vi "NMRvmefull4.vi"() -> ()   [LabVIEW 2013]
uses:
  <vilib>/Utility/file.llb/Read From Spreadsheet File (DBL).vi
  <vilib>/Analysis/NI_AALBase.lvlib
panel:
  in  "Real/quad Q curve":bool=TRUE
  out "Temperature":dbl(graph)=24.5
  out "+3V supply":dbl=3.026 format="%_4g"
  out "Temp (C)":dbl=24.5 format="%_4g"
  in  "RemovePed":bool=TRUE
  in  "IF / LOG Det":bool
  in  "Q curve file":string="realback213.txt"
  out "File name 2":string="C:\\users\\plm\\Desktop\\rssmt\\realback213.txt"
  in  "AutoBaseline":bool=TRUE
  out "RF OK":bool=TRUE
  out "Peak area (V-MHz)":sgl=0.047207057 format="%.5f"
  in  "Gauss Fit":bool=TRUE
  out "NMR Graph + Fit":cluster{cluster{dbl, "Numeric":dbl}[]}[](graph)=[{[{212.6, "Numeric"=-0.00214345238095235}, {212.60999999999999, "Numeric"=0.006892113095217631}, {212.62, "Numeric"=0.0019276785714510206}, {212.63, "Numeric"=0.006363244047621508}, {212.64, "Numeric"=0.006298809523793053}, {212.65, "Numeric"=-0.00026562499997699607}, {212.66, "Numeric"=0.006969940476195022}, {212.67, "Numeric"=0.010905505952368177}, {212.68, "Numeric"=0.009641071428594498}, {212.69, "Numeric"=0.004676636904768078}, {212.7, "Numeric"=0.0005122023809427875}, {212.71, "Numeric"=-0.00015223214283439923}, {212.72, "Numeric"=-0.008416666666659266}, {212.73, "Numeric"=-0.007381101190482957}, {212.74, "Numeric"=-0.0061455357143089286}, {212.75, "Numeric"=0.0058900297619129925}, {212.76, "Numeric"=0.004725595238090845}, {212.77, "Numeric"=0.003161160714266458}, {212.78, "Numeric"=0.0016967261904848666}, {212.79, "Numeric"=0.0038322916666642705}, {212.8, "Numeric"=-0.0059321428571585295}, {212.81, "Numeric"=-0.008196577380943697}, {212.82, "Numeric"=-0.014061011904762707}, {212.82999999999998, "Numeric"=-0.006825446428580642}, {212.84, "Numeric"=-0.0025898809523726522}, {212.85, "Numeric"=-0.002154315476190119}, {212.85999999999999, "Numeric"=0.0002812499999935124}, {212.87, "Numeric"=-0.00438318452380204}, {212.88, "Numeric"=-0.0012476190476179306}, {212.89, "Numeric"=-0.00021205357143272256}, {212.9, "Numeric"=0.009923511904768166}, {212.91, "Numeric"=0.014159077380953854}, {212.92, "Numeric"=0.02259464285714062}, {212.93, "Numeric"=0.036430208333337974}, {212.94, "Numeric"=0.054065773809525215}, {212.95, "Numeric"=0.10650133928571356}, {212.96, "Numeric"=0.20393690476190737}, {212.97, "Numeric"=0.4019724702380962}, {212.98, "Numeric"=0.5035080357142862}, {212.99, "Numeric"=0.42304360119047385}, {213.0, "Numeric"=0.3538791666666667}, {213.01, "Numeric"=0.33051473214285815}, {213.02, "Numeric"=0.2765502976190475}, {213.03, "Numeric"=0.24828586309523684}, {213.04, "Numeric"=0.25662142857142994}, {213.05, "Numeric"=0.24615699404762076}, {213.06, "Numeric"=0.2482925595238066}, {213.07, "Numeric"=0.23562812500000124}, {213.08, "Numeric"=0.19236369047619362}, {213.09, "Numeric"=0.13109925595237593}, {213.1, "Numeric"=0.09613482142857213}, {213.11, "Numeric"=0.07377038690476609}, {213.12, "Numeric"=0.07290595238094486}, {213.13, "Numeric"=0.05124151785714261}, {213.14000000000001, "Numeric"=0.04147708333333814}, {213.15, "Numeric"=0.031812648809513344}, {213.16, "Numeric"=0.03974821428571268}, {213.17000000000002, "Numeric"=0.0409837797619098}, {213.18, "Numeric"=0.030919345238081458}, {213.19, "Numeric"=0.025954910714282364}, {213.2, "Numeric"=0.01839047619048432}, {213.21, "Numeric"=0.01152604166664914}, {213.22, "Numeric"=0.0018616071428516068}, {213.23, "Numeric"=-0.003102827380944837}, {213.24, "Numeric"=-0.003267261904743482}, {213.25, "Numeric"=-0.009831696428579579}, {213.26, "Numeric"=-0.02009613095237444}, {213.27, "Numeric"=-0.017960565476171506}, {213.28, "Numeric"=-0.013825000000011082}, {213.29, "Numeric"=-0.009389434523804457}, {213.3, "Numeric"=-0.005953869047599914}, {213.31, "Numeric"=-0.001018303571443141}, {213.32, "Numeric"=0.0019172619047652106}, {213.33, "Numeric"=-0.018047172619028776}, {213.34, "Numeric"=-0.013611607142875442}, {213.35, "Numeric"=-0.011976041666665615}, {213.36, "Numeric"=-0.012140476190458018}, {213.37, "Numeric"=-0.005904910714308265}, {213.38, "Numeric"=0.0001306547619031248}, {213.39000000000001, "Numeric"=-0.0015337797618877186}, {213.4, "Numeric"=0.002001785714258554}]}, {[{212.6, "Numeric"=4.776893558475571e-16}, {212.60999999999999, "Numeric"=2.4998938518052677e-15}, {212.62, "Numeric"=1.255832331532795e-14}, {212.63, "Numeric"=6.055860163946861e-14}, {212.64, "Numeric"=2.8032001252118955e-13}, {212.65, "Numeric"=1.245565173214598e-12}, {212.66, "Numeric"=5.31267068658366e-12}, {212.67, "Numeric"=2.1751710942402627e-11}, {212.68, "Numeric"=8.548856700490645e-11}, {212.69, "Numeric"=3.225200648435985e-10}, {212.7, "Numeric"=1.1679910816561408e-09}, {212.71, "Numeric"=4.0602839092061546e-09}, {212.72, "Numeric"=1.3549003796765097e-08}, {212.73, "Numeric"=4.3400268270931275e-08}, {212.74, "Numeric"=1.3344784063174184e-07}, {212.75, "Numeric"=3.938807665763447e-07}, {212.76, "Numeric"=1.1159688835032996e-06}, {212.77, "Numeric"=3.0351033450249673e-06}, {212.78, "Numeric"=7.923717225927055e-06}, {212.79, "Numeric"=1.9857224263191096e-05}, {212.8, "Numeric"=4.77685655501104e-05}, {212.81, "Numeric"=0.00011030620579413602}, {212.82, "Numeric"=0.00024450727185348263}, {212.82999999999998, "Numeric"=0.0005202567224041215}, {212.84, "Numeric"=0.001062619321376955}, {212.85, "Numeric"=0.00208339589052297}, {212.85999999999999, "Numeric"=0.003921028375121005}, {212.87, "Numeric"=0.00708373415515426}, {212.88, "Numeric"=0.012284531843177892}, {212.89, "Numeric"=0.020449799470303114}, {212.9, "Numeric"=0.03267785821490993}, {212.91, "Numeric"=0.05012474792628662}, {212.92, "Numeric"=0.07380485072971074}, {212.93, "Numeric"=0.10431618549469776}, {212.94, "Numeric"=0.141531326388596}, {212.95, "Numeric"=0.1843264006586668}, {212.96, "Numeric"=0.23043932570196038}, {212.97, "Numeric"=0.27654113177117073}, {212.98, "Numeric"=0.318564196067707}, {212.99, "Numeric"=0.35226401239535293}, {213.0, "Numeric"=0.37391568130834746}, {213.01, "Numeric"=0.3809896410966228}, {213.02, "Numeric"=0.37263765937905063}, {213.03, "Numeric"=0.3498600920751344}, {213.04, "Numeric"=0.3153088466879908}, {213.05, "Numeric"=0.2727796658425095}, {213.06, "Numeric"=0.22652801382782384}, {213.07, "Numeric"=0.18057845310601628}, {213.08, "Numeric"=0.13817963040978265}, {213.09, "Numeric"=0.10149770261945476}, {213.1, "Numeric"=0.07156529811815136}, {213.11, "Numeric"=0.048437625424841466}, {213.12, "Numeric"=0.031470039729766065}, {213.13, "Numeric"=0.019626634059215383}, {213.14000000000001, "Numeric"=0.011749745126604191}, {213.15, "Numeric"=0.006752197770040614}, {213.16, "Numeric"=0.003724739884438077}, {213.17000000000002, "Numeric"=0.001972335681903894}, {213.18, "Numeric"=0.0010025355948645779}, {213.19, "Numeric"=0.0004891621640607406}, {213.2, "Numeric"=0.00022910786660302744}, {213.21, "Numeric"=0.00010300569388837138}, {213.22, "Numeric"=4.445458393558479e-05}, {213.23, "Numeric"=1.8416451552346927e-05}, {213.24, "Numeric"=7.3236814655574865e-06}, {213.25, "Numeric"=2.795677209790716e-06}, {213.26, "Numeric"=1.0244215183627779e-06}, {213.27, "Numeric"=3.6033333878935025e-07}, {213.28, "Numeric"=1.2166461504331838e-07}, {213.29, "Numeric"=3.9432854284808336e-08}, {213.3, "Numeric"=1.2268352014433039e-08}, {213.31, "Numeric"=3.663939808945258e-09}, {213.32, "Numeric"=1.0503753455418787e-09}, {213.33, "Numeric"=2.8905121249409887e-10}, {213.34, "Numeric"=7.635529486391247e-11}, {213.35, "Numeric"=1.93614379589947e-11}, {213.36, "Numeric"=4.712703817908686e-12}, {213.37, "Numeric"=1.1011253745842512e-12}, {213.38, "Numeric"=2.469661789025322e-13}, {213.39000000000001, "Numeric"=5.3170688138188436e-14}, {213.4, "Numeric"=1.0988569689482739e-14}]}]
  in  "Amp of Q curve":dbl=3.0 min=0.0 max=7.0 step=0.01 format="%_3f"
  in  "Subtract Q curve":bool=TRUE
  in  "Adjust Tune":bool
  out "Ped Offset":dbl(graph)=0.005645833333333402
  out "Pedestal Difference":dbl(graph)=0.06520833333333734
  out "# Good Spectra":i32=977
  in  "Quality cuts":bool=TRUE
  out "Pedestal OK":bool=TRUE
  out "Sweep #":i32=3604
  out "1st Sweep":bool
  out "ADC volts OK":bool=TRUE
  out "Peak Height Distribution":cluster{"Y":dbl[], "Y":dbl[]}[](graph)=[{"Y"=[0.36242839752414713, 0.3626627543764223, 0.36289711122869756, 0.3631314680809728, 0.363365824933248, 0.3636001817855232, 0.36383453863779847, 0.36406889549007365, 0.3643032523423489, 0.3645376091946241, 0.3647719660468993, 0.36500632289917456, 0.36524067975144975, 0.365475036603725, 0.3657093934560002, 0.3659437503082754, 0.36617810716055066, 0.36641246401282584, 0.3666468208651011, 0.36688117771737633, 0.3671155345696515, 0.36734989142192676, 0.36758424827420194, 0.3678186051264772, 0.3680529619787524, 0.3682873188310276, 0.36852167568330285, 0.3687560325355781, 0.3689903893878533, 0.3692247462401285, 0.3694591030924037, 0.36969345994467895, 0.3699278167969542, 0.3701621736492294, 0.3703965305015046, 0.37063088735377986, 0.37086524420605504, 0.3710996010583303, 0.37133395791060547, 0.3715683147628807, 0.37180267161515596, 0.37203702846743114, 0.3722713853197064, 0.37250574217198157, 0.3727400990242568, 0.37297445587653205, 0.37320881272880724, 0.3734431695810825, 0.3736775264333577, 0.3739118832856329, 0.37414624013790815, 0.37438059699018333, 0.3746149538424586, 0.3748493106947338, 0.375083667547009, 0.37531802439928424, 0.3755523812515595, 0.37578673810383467, 0.3760210949561099, 0.3762554518083851, 0.37648980866066034, 0.3767241655129356, 0.37695852236521077, 0.377192879217486, 0.3774272360697612, 0.37766159292203644, 0.3778959497743117, 0.37813030662658687, 0.3783646634788621, 0.37859902033113735, 0.37883337718341253, 0.3790677340356878, 0.37930209088796296, 0.3795364477402382, 0.37977080459251344, 0.38000516144478863, 0.38023951829706387, 0.3804738751493391, 0.3807082320016143, 0.38094258885388954, 0.3811769457061647, 0.38141130255843997, 0.3816456594107152, 0.3818800162629904, 0.38211437311526564, 0.3823487299675409, 0.38258308681981607, 0.3828174436720913, 0.3830518005243665, 0.38328615737664173, 0.383520514228917, 0.38375487108119216, 0.3839892279334674, 0.3842235847857426, 0.38445794163801783, 0.38469229849029307, 0.38492665534256826, 0.3851610121948435, 0.38539536904711874, 0.3856297258993939], "Y"=[1.0, 0.0, 2.0, 1.0, 3.0, 3.0, 2.0, 1.0, 2.0, 4.0, 0.0, 3.0, 4.0, 3.0, 4.0, 2.0, 3.0, 6.0, 4.0, 4.0, 4.0, 6.0, 11.0, 6.0, 7.0, 6.0, 8.0, 8.0, 6.0, 13.0, 10.0, 12.0, 14.0, 27.0, 14.0, 15.0, 23.0, 16.0, 16.0, 12.0, 13.0, 24.0, 23.0, 17.0, 28.0, 22.0, 18.0, 20.0, 25.0, 21.0, 25.0, 21.0, 24.0, 16.0, 27.0, 16.0, 18.0, 13.0, 18.0, 23.0, 20.0, 19.0, 7.0, 13.0, 16.0, 12.0, 20.0, 15.0, 13.0, 13.0, 9.0, 13.0, 11.0, 10.0, 6.0, 4.0, 10.0, 5.0, 9.0, 6.0, 3.0, 5.0, 5.0, 3.0, 4.0, 3.0, 3.0, 3.0, 3.0, 1.0, 4.0, 2.0, 3.0, 1.0, 1.0, 1.0, 1.0, 1.0, 0.0, 1.0]}]
  in  "# of Sweeps":i32=10000
  out "Std Dev (V)":dbl=0.004257288736008398 format="%_2g"
  out "Peak mean (V)":dbl=0.37397306272927033 format="%_4g"
  out "Peak Height":dbl(graph)=0.38100328829507124
  in  "Raw Data":bool=TRUE
  in  "Tank RF":bool=TRUE
  in  "IF Atten (dB)":i8 min=0 max=31 step=1
  in  "IFoffset (V)":dbl=-2.0905283999999975 min=-4.0 max=4.0 step=0.001 format="%.4f"
  in  "Tune  (V)":dbl=0.6128999999999999 min=0.0 max=5.0 step=0.001 format="%.4f"
  in  "Hi / Lo IF Gain":bool
  out "Voltage Array":sgl[](array[numeric])=[0.449, 0.4352, 0.408, 0.3908, 0.3697, 0.3427, 0.3301, 0.3148, 0.2949, 0.2719, 0.2503, 0.2328, 0.2083, 0.1937, 0.1799, 0.1775, 0.1625, 0.1477, 0.1336, 0.1237, 0.1025, 0.0894, 0.0733, 0.0709, 0.0661, 0.0581, 0.0527, 0.0408, 0.0373, 0.0323, 0.037, 0.0364, 0.0406, 0.0508, 0.0654, 0.1154, 0.211, 0.4078, 0.5087, 0.4282, 0.3596, 0.3374, 0.2852, 0.2593, 0.2706, 0.2637, 0.27, 0.2621, 0.2242, 0.1689, 0.1405, 0.1253, 0.1322, 0.1189, 0.1181, 0.118, 0.1361, 0.1481, 0.1494, 0.1564, 0.1614, 0.1677, 0.1718, 0.1812, 0.196, 0.205, 0.2109, 0.2298, 0.2513, 0.2737, 0.2957, 0.3198, 0.3425, 0.3429, 0.3683, 0.3915, 0.4135, 0.4425, 0.4719, 0.4942, 0.5223] format="%.4f"
  in  "Invert Polarity":bool
  out "Pedestal Diff (V)":sgl=0.06520833 format="%.3f"
  out "Peak amp (V)":sgl=0.3810033 format="%.3f"
  in  "Save Data to File":bool
  in  "RF Level (dBm)":dbl=-1.0 min=-10.0 max=1.0 step=0.1 format="%.2f"
  out "SMT error out":errorcluster
  out "Sample RMS (V)":dbl=0.016388888888888887 format="%.4f"
  in  "# Sample/step":i32=200 min=1 max=1000 step=100
  in  "Step Width (MHz)":dbl=0.01 min=0.0 max=1000.0 step=0.0005 format="%.4f"
  in  "Freq Span (MHz)":dbl=0.8 min=0.0 max=3000.0 step=0.1 format="%.3f"
  in  "Center Freq (MHz)":dbl=213.0 min=0.005 max=6000.0 step=0.1 format="%.3f"
  in  "Sweep Mode":u16(ring)=3 items=["Off", "Single", "Auto", "Step"]
  in  "GPIB Addr (28)":refnum<visa-resource-name>="GPIB0::28::INSTR"
  # "E1039 Prototype NMR Control Panel"
  # "Settings"
  # "D\nA\nC"
  # "R\nF\n\nG\nE\nN \n\n+\n\nI\nF"
  # "A\nD\nC"
  # "D\nA\nT\nA\n\n+\n\nA \nN\nA\nL\nY\nS\nI\nS"
  # "I\n/\nO"
  # "Results"
  # "A\nv\ne\nr\na\ng\ne"
  # "S\nw\ne\ne\np"
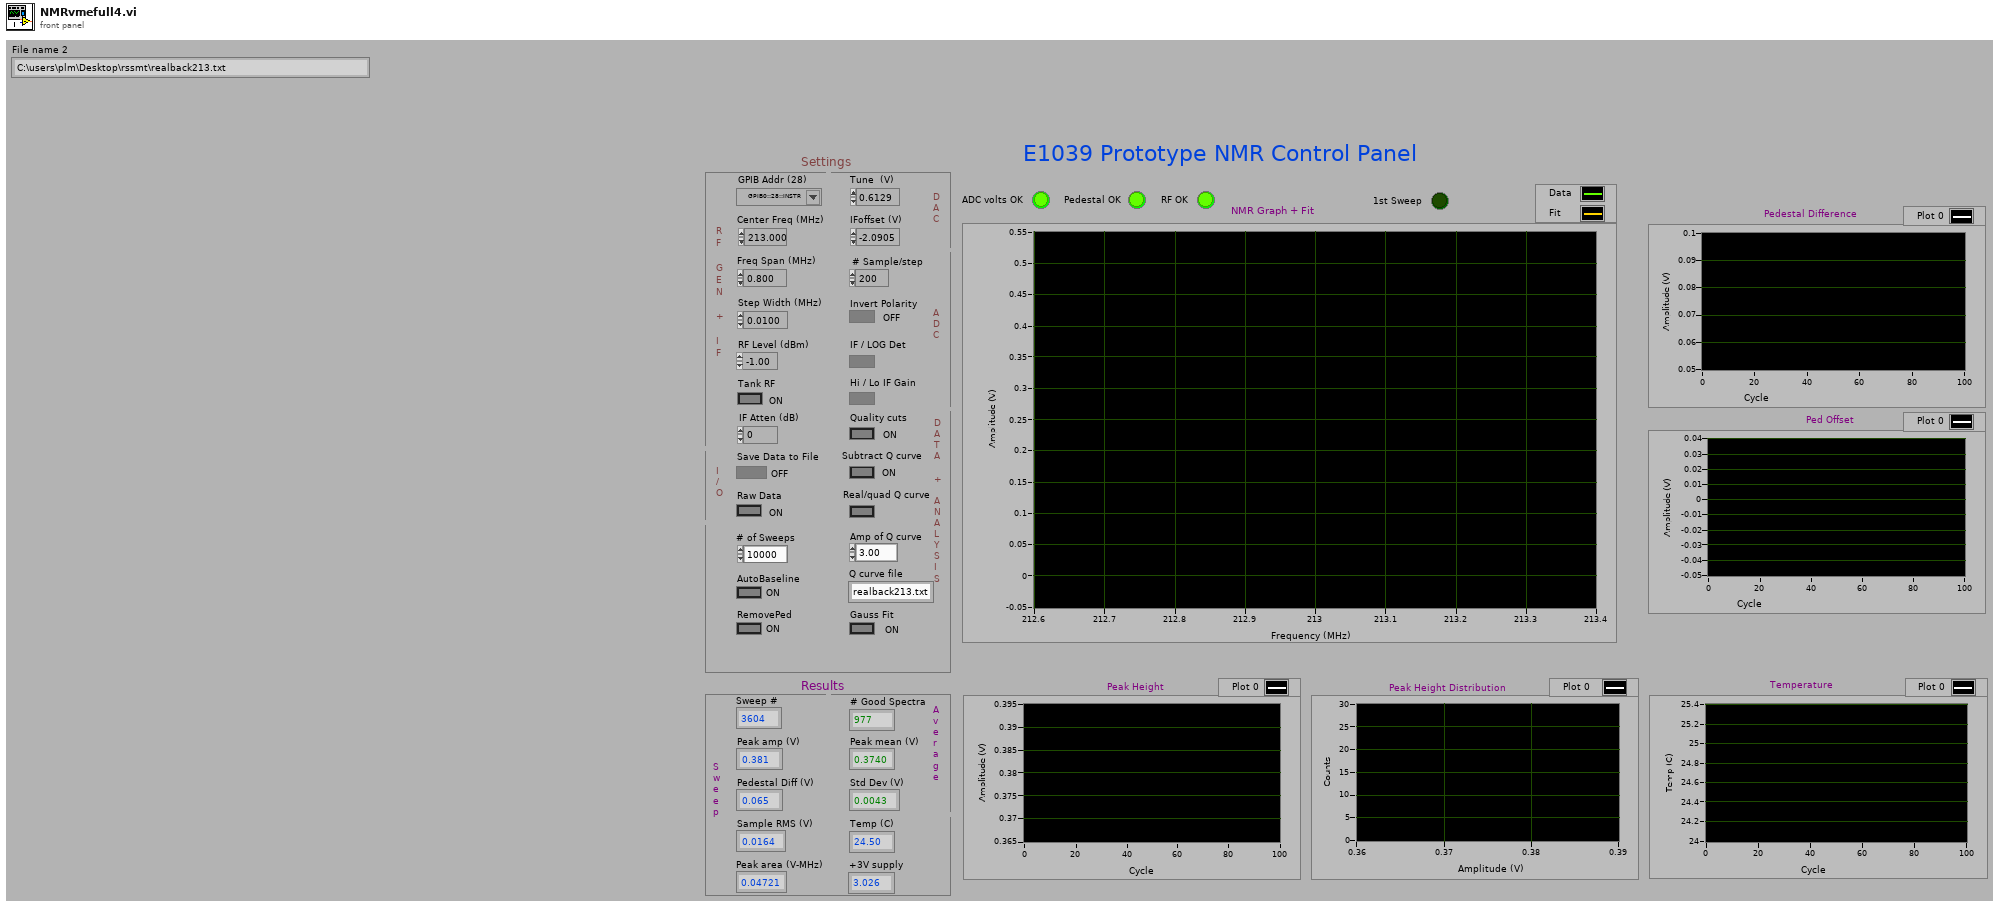
[diagram p1: front panel]
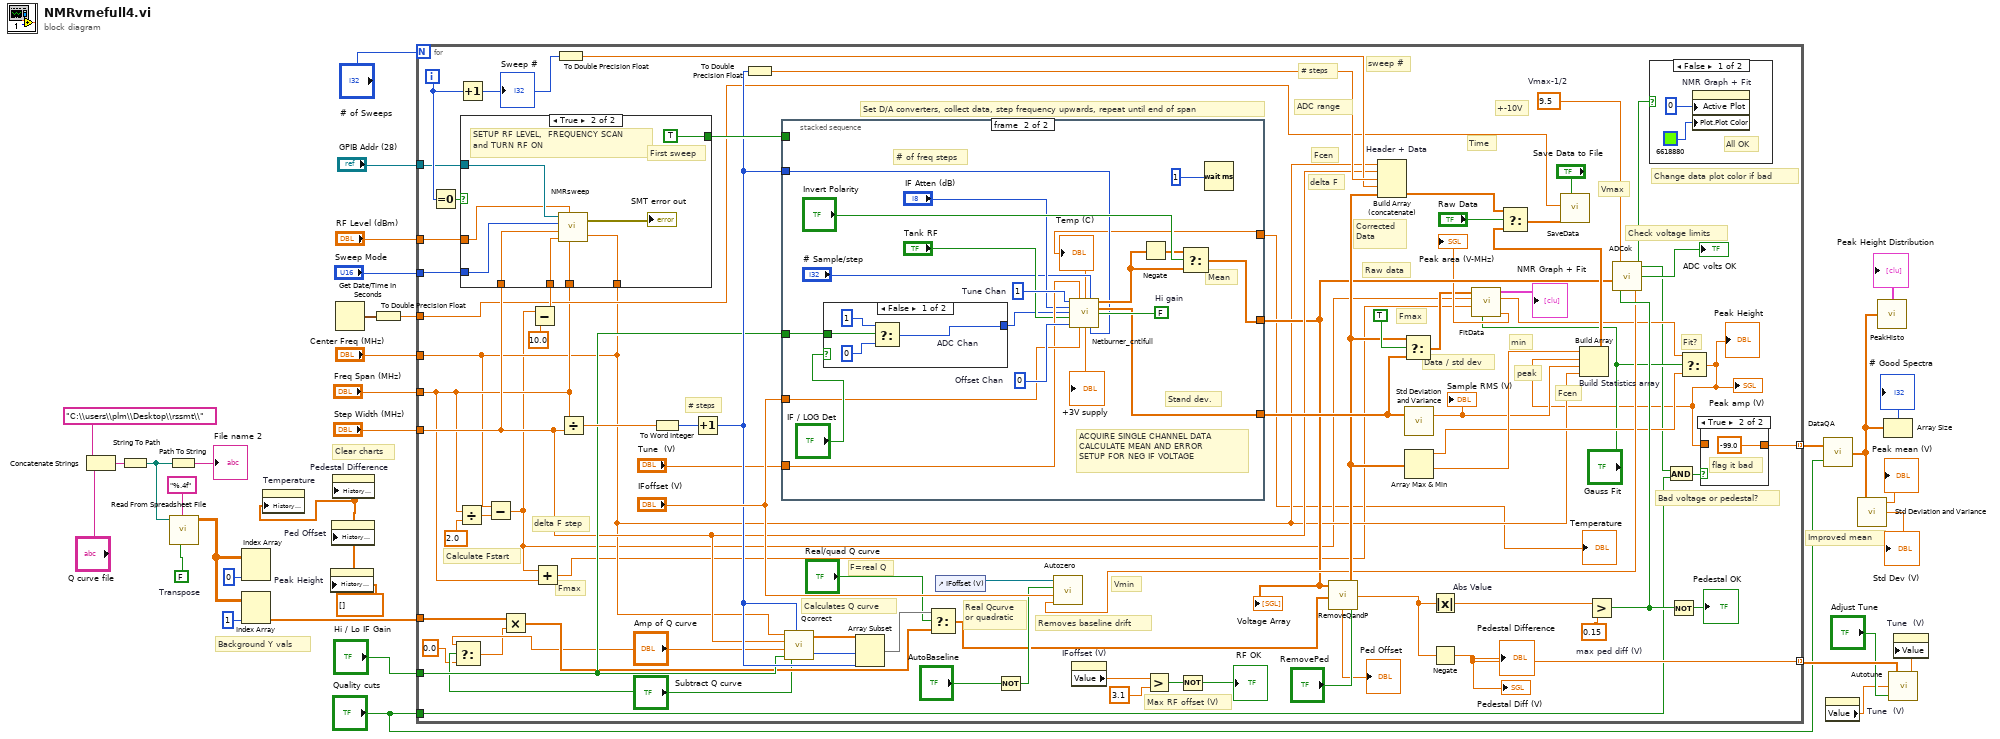
[diagram p0: block diagram]
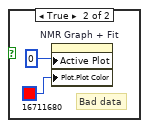
[diagram p2: hidden frame]
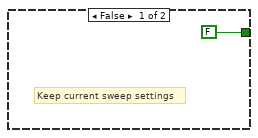
[diagram p4: hidden frame]
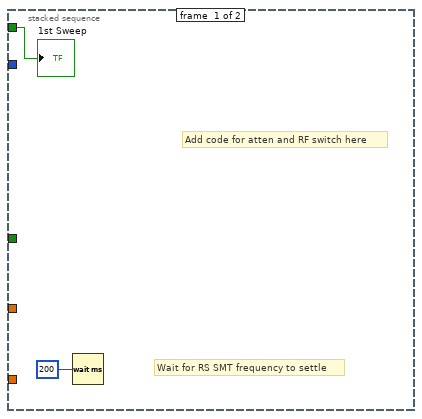
[diagram p5: hidden frame]
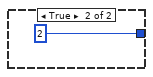
[diagram p6: hidden frame]
diagram:
  w9 = FALSE  # Transpose
  w1 = dbl[] []
  # "Background Y vals"
  # "Clear charts"
  # "Improved mean"
  n1 = Concatenate Strings "Concatenate Strings"("C:\\users\\plm\\Desktop\\rssmt\\", "Q curve file") -> (w12:string)
  n2 = String To Path(string=w12) -> (path=w8:path)
  n3 = Path To String(path=w8) -> (string=→"File name 2":string)
  n4 = call-poly <vilib>:"Read From Spreadsheet File.vi"("transpose (no:F)"=w9, "format (%.3f)"="%.4f", "file path (dialog if empty)"=w8) -> ("all rows"=w7:dbl[][])  [unwired: 4 in, 4 out]
  n5 = Index Array "Index Array"(array=w7, index (col)=0) -> ()  [unwired: 1 in, 1 out]
  n6 = Index Array(array=w7, index (col)=1) -> (element=w2:dbl[])  [unwired: 1 in]
  n7 = property on="Temperature" class="WFChart (strict)"("History Data"=w1) -> ()  [unwired: 2 in, 2 out]
  n8 = property on="Peak Height" class="WFChart (strict)"("History Data"=w1) -> ()  [unwired: 2 in, 2 out]
  n9 = property on="Ped Offset" class="WFChart (strict)"("History Data"=w1) -> ()  [unwired: 2 in, 2 out]
  n10 = property on="Pedestal Difference" class="WFChart (strict)"("History Data"=w1) -> ()  [unwired: 2 in, 2 out]
  n11 = Get Date/Time In Seconds() -> (seconds since 1Jan1904=w14:timestamp)
  n12 = To Double Precision Float(number=w14) -> (double precision float=w13:dbl)
  n13 = for {
    N: "# of Sweeps" -> [_]
    tunnel: [w94] -> w29 mode=indexing
    tunnel: "Quality cuts" -> [w71]
    tunnel: [w77] -> w26 mode=indexing
    tunnel: "Center Freq (MHz)" -> [w58]
    tunnel: "Freq Span (MHz)" -> [w64]
    tunnel: "Step Width (MHz)" -> [w70]
    tunnel: "Sweep Mode" -> [w81]
    tunnel: "Hi / Lo IF Gain" -> [w80]
    tunnel: "GPIB Addr (28)" -> [w79]
    tunnel: "RF Level (dBm)" -> [w78]
    tunnel: w13 -> [w65]
    tunnel: w2 -> [w43]
    i -> [w92]
    w75 = 9.5  # Vmax-1/2
    w95 = 0.15  # max ped diff (V)
    # "F=real Q"
    # "Real Qcurve\nor quadratic"
    # "+-10V"
    # "Vmax"
    # "Change data plot color if bad"
    # "Max RF offset (V)"
    # "Fmax"
    # "Fit?"
    # "Fmax"
    # "Time"
    # "Vmin"
    # "min"
    # "peak"
    # "Raw data"
    # "Corrected\nData"
    # "Fcen"
    # "delta F"
    # "# steps"
    # "ADC range"
    # "sweep #"
    # "Fcen"
    # "Set D/A converters, collect data, step frequency upwards, repeat until end of span"
    # "Calculates Q curve"
    # "Removes baseline drift"
    # "Bad voltage or pedestal?"
    # "Check voltage limits"
    # "Data / std dev"
    # "# steps"
    # "Calculate Fstart"
    # "delta F step"
    n14 = Equal To 0?(x=w92) -> (x = 0?=w97:bool)
    n15 = Select(t="Amp of Q curve", s="Subtract Q curve", f=0.0) -> (s? t:f=w38:dbl)
    n16 = Divide(x=w64, y=sgl 2.0) -> (x/y=w108:dbl)
    n17 = Increment(x=w92) -> (x+1=w82:i32)
    "Sweep #" <- w82
    n18 = Subtract(x=w58, y=w108) -> (x-y=w53:dbl)
    n19 = Multiply(x=w43, y=w38) -> (x*y=w42:dbl[])
    n20 = Subtract(x=w53, y=10.0) -> (x-y=w106:dbl)
    n21 = case shown="True" w97 {
      tunnel: w106 -> [_ w126]
      tunnel: w70 -> [_ w124]
      tunnel: w58 -> [_ w123]
      tunnel: w64 -> [_ w125]
      tunnel: [FALSE TRUE] -> w96
      tunnel: w81 -> [_ w120]
      tunnel: w79 -> [_ w119]
      tunnel: w78 -> [_ w118]
      frame False {
        # "Keep current sweep settings"
      }
      frame True {
        # "First sweep"
        # "SETUP RF LEVEL,  FREQUENCY SCAN\nand TURN RF ON"
        n22 = call "NMRsweep.vi"("Center Freq (MHz)"=w123, "Freq Span (MHz)"=w125, "RF Level (dBm)"=w118, "Foffset (MHz)"=w126, "Step Width (MHz)"=w124, "Sweep Mode"=w120, "GPIB Addr (28)"=w119) -> ("error out"=→"SMT error out":errorcluster)
      }
    }
    n23 = Add(x=w53, y=w64) -> (x+y=w52:dbl)
    n24 = To Double Precision Float(number=w82) -> (double precision float=w83:dbl)
    n25 = Divide(x=w64, y=w70) -> (x/y=w110:dbl)
    n26 = To Word Integer(number=w110) -> (16bit integer=w107:i16)
    n27 = Increment(x=w107) -> (x+1=w86:i16)
    n28 = To Double Precision Float(number=w86) -> (double precision float=w85:dbl)
    n29 = stacked-sequence {
      tunnel: [_ w134] -> w100
      tunnel: [_ w146] -> w68
      tunnel: w86 -> [_ w131]
      tunnel: "IFoffset (V)" -> [_ w141]
      tunnel: w80 -> [_ w144]
      tunnel: w96 -> [w127 _]
      tunnel: "Tune  (V)" -> [_ w139]
      tunnel: [_ w129] -> w34
      frame #0 {
        # "Add code for atten and RF switch here"
        # "Wait for RS SMT frequency to settle"
        n30 = Wait (ms)(milliseconds to wait=200) -> ()  [unwired: 1 out]
        "1st Sweep" <- w127
      }
      frame #1 {
        w136 = FALSE  # Hi gain
        w142 = 0  # Offset Chan
        w140 = 1  # Tune Chan
        # "Stand dev."
        # "Mean"
        # "ACQUIRE SINGLE CHANNEL DATA\nCALCULATE MEAN AND ERROR\nSETUP FOR NEG IF VOLTAGE"
        # "# of freq steps"
        n31 = case shown="False" "IF / LOG Det" {
          tunnel: w144 -> [w152 _]
          tunnel: [w149 2] -> w133
          frame False {
            n32 = Select "ADC Chan"(t=1, s=w152, f=0) -> (s? t:f=w149:i32)
          }
          frame True {
          }
        }
        n33 = call "Netburner_cntlfull.vi"("Tune DAC"=w140, "Tune Volt"=w139, "# Data"="# Sample/step", "IF Atten (dB)"="IF Atten (dB)", "NMR ADC"=w133, "Hi Gain"=w136, "Tank RF"="Tank RF", "Offset DAC"=w142, "Offset Volt"=w141, "# f steps"=w131) -> ("Temp (C)"=w129:dbl, "ADC value"=w135:dbl[], "ADC error"=w134:dbl[], "Volts"=→"+3V supply":dbl)  [unwired: 2 out]
        "Temp (C)" <- w129
        n34 = Negate(x=w135) -> (-x=w145:dbl[])
        n35 = Select(t=w145, s="Invert Polarity", f=w135) -> (s? t:f=w146:dbl[])
        n36 = Wait (ms)(milliseconds to wait=1) -> ()  [unwired: 1 out]
      }
    }
    "Voltage Array" <- w68
    "Temperature" <- w34
    n37 = call "Qcorrect.vi"("Subtract Q curve"="Subtract Q curve", "Nstep"=w86, "IF or Log"=w80, "Amp of Q curve"="Amp of Q curve", "Step Width (MHz)"=w70, "Center Freq (MHz)"=w58) -> ("Start"=w101:i32, "Array"=w102:dbl[])
    n38 = Array Subset "Array Subset"(array=w102, index=w101, length=w86) -> (w46:dbl[])
    n39 = Select(t=w46, s="Real/quad Q curve", f=w42) -> (s? t:f=w45:dbl[])
    n40 = control-ref of="IFoffset (V)"() -> (w74:refnum<vi>)
    n41 = Not(x="AutoBaseline") -> (.not. x?=w47:bool)
    n42 = property on="IFoffset (V)" class="DigNum (strict)"() -> ("Value"=w62:dbl)  [unwired: 2 in, 2 out]
    n43 = Greater?(x=w62, y=3.1) -> (0:w60:bool)
    n44 = Not(x=w60) -> (.not. x?=→"RF OK":bool)
    n45 = call "RemoveQandP.vi"("Subtract Ped?"="RemovePed", "Qcurve"=w45, "Raw data"=w68) -> ("Ped L-R"=w88:dbl, "Corrected data"=w84:dbl[], "Ped Offfset"=→"Ped Offset":dbl)
    n46 = Build Array (concatenate) "Header + Data"(w58, w70, w85, w83, w84) -> (w87:dbl[])
    n47 = Select(t=w84, s=TRUE, f=w100) -> (s? t:f=w54:dbl[])
    n48 = call <vilib>:"Std Deviation and Variance.vi"("X"=w100) -> ("mean"=w69:dbl)  [unwired: 1 in, 2 out]
    "Sample RMS (V)" <- w69
    n49 = Array Max & Min(array=w84) -> (max value=w63:dbl, min value=w99:dbl)  [unwired: 2 out]
    n50 = Absolute Value "Abs Value"(x=w88) -> (abs(x)=w90:dbl)
    n51 = Negate(x=w88) -> (-x=w77:dbl)
    "Pedestal Diff (V)" <- w77
    "Pedestal Difference" <- w77
    n52 = call "FitData.vi"("Fit?"="Gauss Fit", "Fmax"=w52, "Fmin"=w53, "Yarray"=w54) -> ("Peak Area (V-MHz)"=→"Peak area (V-MHz)":dbl, "Amplitude (V)"=w56:dbl, "NMR Graph + Fit"=→"NMR Graph + Fit":cluster{cluster{dbl, "Numeric":dbl}[]}[])  [unwired: 2 out]
    n53 = Greater?(x=w90, y=w95) -> (0:w76:bool)
    n54 = call "ADCok.vi"("PedOK"=w76, "Array"=w68, "Vmax-1/2"=w75) -> ("Vmin"=w73:dbl, "ADC voltages OK"=→"ADC volts OK":bool, "Allok"=w50:bool)
    n55 = call "Autozero.vi"("Vmin (V)"=w73, "IFoffset (V)"="IFoffset (V)", "IF or Log"=w47, "reference"=w74) -> ()
    n56 = case shown="False" w50 {
      frame False {
        # "All OK"
        n57 = property on="NMR Graph + Fit" class="XYGraph (strict)"("Active Plot"=0, "Plot.Plot Color"=u32 6618880) -> ()  [unwired: 2 in, 2 out]
      }
      frame True {
        # "Bad data"
        n58 = property on="NMR Graph + Fit" class="XYGraph (strict)"("Active Plot"=0, "Plot.Plot Color"=u32 16711680) -> ()  [unwired: 2 in, 2 out]
      }
    }
    n59 = And(x=w50, y=w71) -> (x .and. y?=w91:bool)
    n60 = Not(x=w76) -> (.not. x?=→"Pedestal OK":bool)
    n61 = Select(t=w56, s="Gauss Fit", f=w63) -> (s? t:f=w49:dbl)
    "Peak amp (V)" <- w49
    "Peak Height" <- w49
    n62 = Build Array "Build Statistics array"(w99, w49, w69, w58) -> (w105:dbl[])
    n63 = Select(t=w87, s="Raw Data", f=w105) -> (s? t:f=w66:dbl[])
    n64 = call "SaveData.vi"("Array"=w66, "Save Data to File"="Save Data to File", "Ext time (sec)"=w65) -> ()  [unwired: 1 out]
    n65 = case shown="True" w91 {
      tunnel: [w115 -99.0] -> w94
      tunnel: w49 -> [w115 _]
      frame False {
        # "Data OK"
      }
      frame True {
        # "flag it bad"
      }
    }
  }
  n66 = call "DataQA.vi"("Quality cuts"="Quality cuts", "Data In"=w29) -> ("Data Out"=w28:dbl[])
  n67 = property on="Tune  (V)" class="DigNum (strict)"() -> ("Value"=w17:dbl)  [unwired: 2 in, 2 out]
  n68 = call <vilib>:"Std Deviation and Variance.vi"("X"=w28) -> ("mean"=→"Peak mean (V)":dbl, "standard deviation"=→"Std Dev (V)":dbl)  [unwired: 1 in, 1 out]
  n69 = call "PeakHisto.vi"("Data Out"=w28) -> ("XY Graph"=→"Peak Height Distribution":cluster{"Y":dbl[], "Y":dbl[]}[])
  n70 = Array Size(array=w28) -> (size(s)=→"# Good Spectra":i32)
  n71 = call "Autotune.vi"("Adjust Tune"="Adjust Tune", "Tune Vin"=w17, "Pedestal Diff"=w26) -> ("Tune Vout"=w16:dbl)
  n72 = property on="Tune  (V)" class="DigNum (strict)"("Value"=w16) -> ()  [unwired: 2 in, 2 out]
